vi "load_ltrace.vi"(7 "Progress":refnum<vi>, 8 "error in":errorcluster, 10 "File path":path) -> (0 "error out":errorcluster, 2 "File index":T1[](array[typedef]) {"Timestamp" format="%<%.3X>T"}, 4 "Out of order":i32, 5 "Flag names":string[](array[string]), 6 "Missing":i32)   [LabVIEW 2013]
uses:
  ltrace_index.ctl
panel:
  # "Sequence number checking"
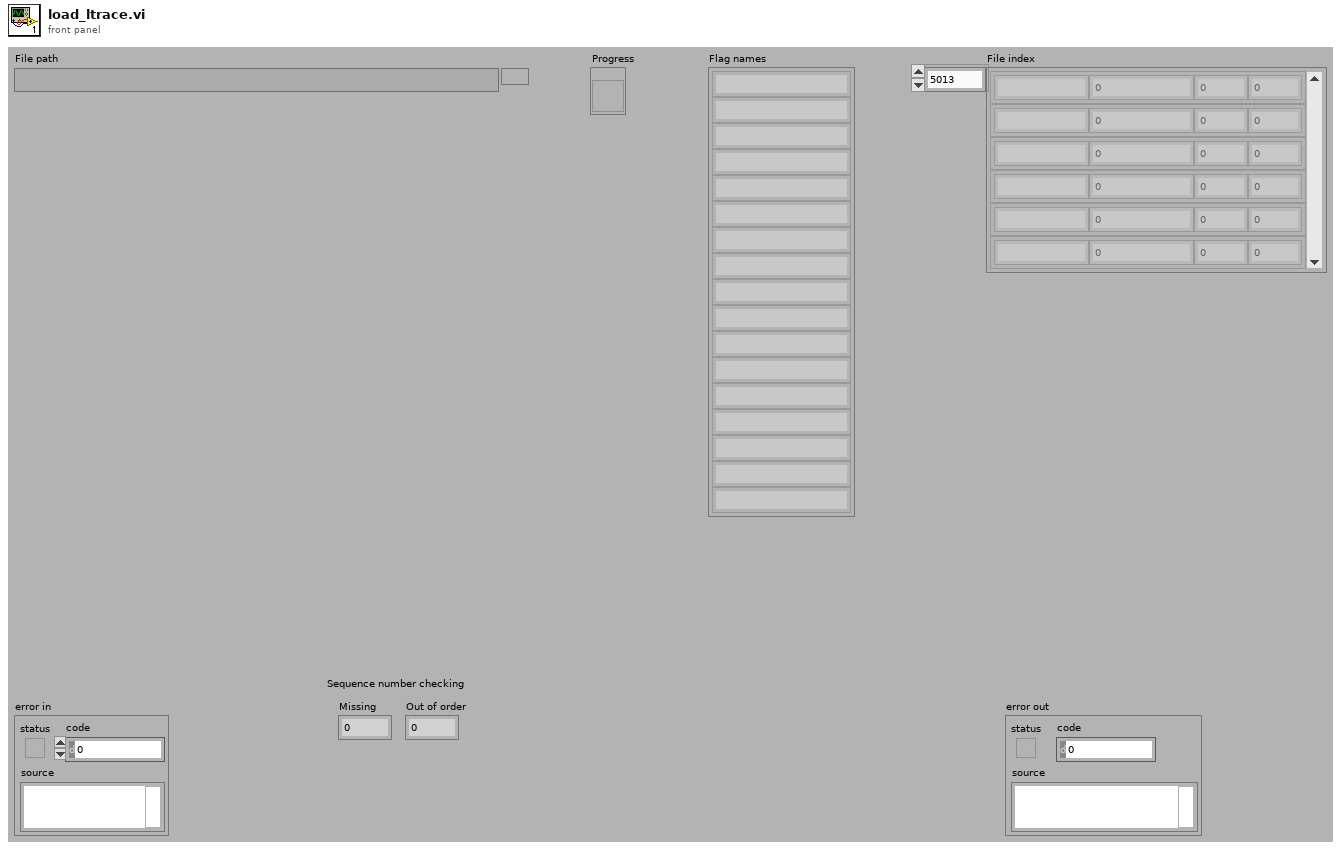
[diagram p1: front panel]
types:
  T1 = typedef "ltrace_index.ctl" = cluster{"Timestamp":timestamp, "Offset":i64, "Sequence":u32, "Flags":u32}
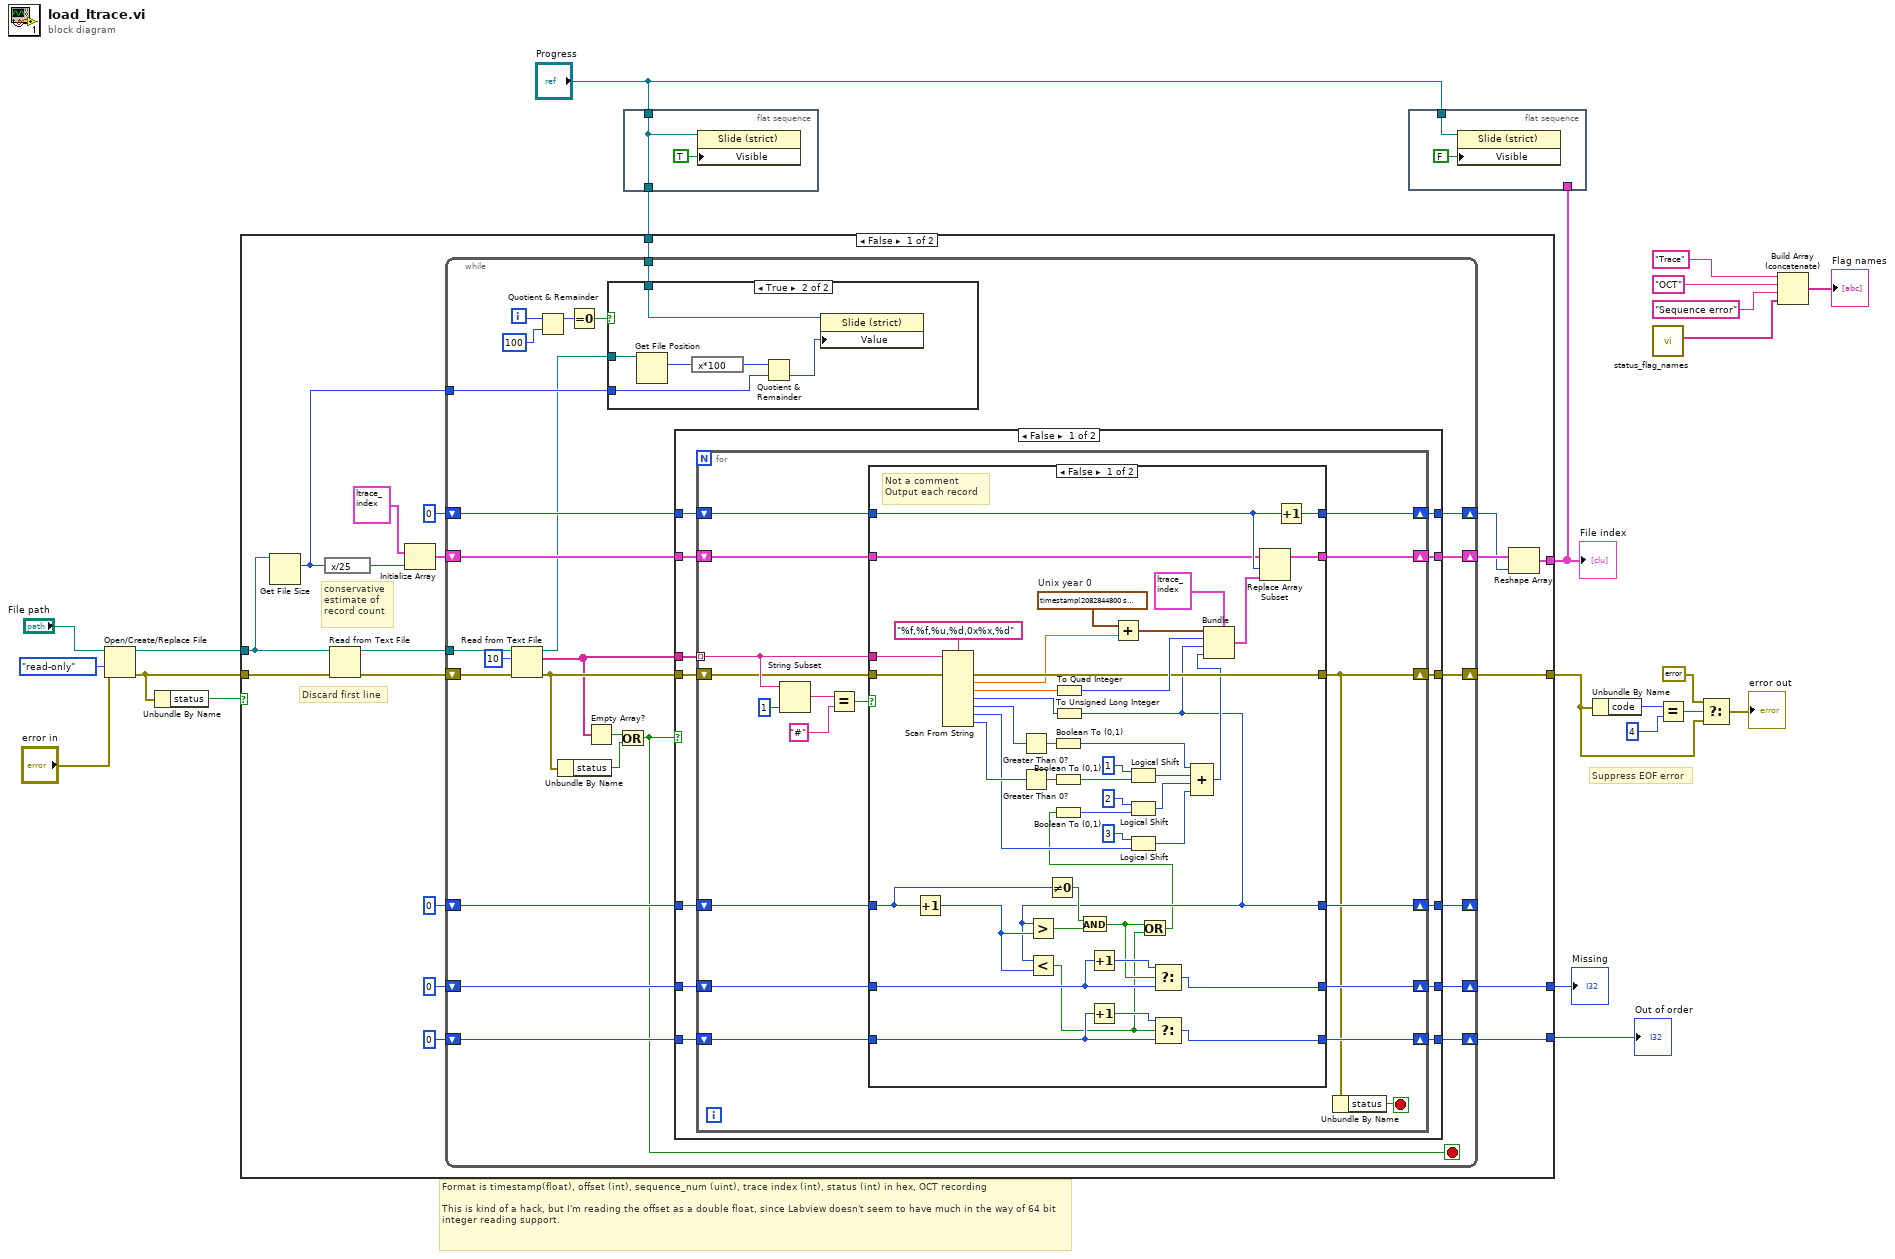
[diagram p0: block diagram]
diagram:
  # "Suppress EOF error"
  # "Format is timestamp(float), offset (int), sequence_num (uint), trace index (int), status (int) in hex, OCT recording\n\nThis is kind of a hack, but I'm reading the offset as a double float, since Labview doesn't seem to have much in the way of 64 bit integer reading support."
  n1 = Open/Create/Replace File(file path (use dialog)="File path", error in="error in", access (0:read/write)=enum16{"read/write", "read-only", "write-only"}."read-only") -> (refnum out=w14:refnum<file>, error out=w19:errorcluster)  [unwired: 3 in, 1 out]
  n2 = Unbundle By Name(w19) -> ("status"=w20:bool)
  n3 = case shown="False" w20 {
    tunnel: w19 -> [w25 w162]
    tunnel: w14 -> [w26 _]
    tunnel: [w33 _] -> w1
    tunnel: [w32 _] -> w2
    tunnel: [w31 _] -> w15
    tunnel: w17 -> [w29 _]
    tunnel: [w27 w162] -> w10
    frame False {
      # "Discard first line"
      # "conservative\nestimate of \nrecord count"
      n4 = Get File Size(file=w26) -> (size (in bytes)=w28:i64)  [unwired: 1 in, 2 out]
      n5 = expression code="x/25"(w28) -> (w30:i64)
      n6 = Read from Text File(file (use dialog)=w26, error in=w25) -> (refnum out=w23:refnum<file>, error out=w24:errorcluster)  [unwired: 2 in, 2 out]
      n7 = Initialize Array(T1 {"Timestamp"=timestamp(0 s since 1904-01-01), "Offset"=0, "Sequence"=0, "Flags"=0} ("output cluster"), w30) -> (w41:T1[])
      n8 = while {
        shift-right: [w58] -> w39
        shift-left: w41 -> [w59]
        shift-right: [w66] -> w38
        shift-left: 0 ("output 3") -> [w67]
        shift-right: [w65] -> _
        shift-left: u32 0 ("unsigned 32bit integer") -> [w64]
        shift-right: [w60] -> w32
        shift-left: 0 ("output 5") -> [w63]
        shift-right: [w61] -> w33
        shift-left: 0 ("output 5") -> [w62]
        tunnel: w29 -> [w56]
        tunnel: w28 -> [w55]
        tunnel: w23 -> [w54]
        shift-right: [w51] -> w27
        shift-left: w24 -> [w53]
        i -> [w57]
        stop <- w46 stop-if-true
        n9 = Read from Text File(file (use dialog)=w54, count=10, error in=w53) -> (refnum out=w42:refnum<file>, text=w49:string[], error out=w52:errorcluster)  [unwired: 1 in, 1 out]
        n10 = Quotient & Remainder(x=w57, y=100) -> (x-y*floor(x/y)=w43:i32)  [unwired: 1 out]
        n11 = Unbundle By Name(w52) -> ("status"=w47:bool)
        n12 = Equal To 0?(x=w43) -> (x = 0?=w44:bool)
        n13 = Empty Array?(array=w49) -> (empty?=w48:bool)
        n14 = case shown="True" w44 {
          tunnel: w56 -> [_ w73]
          tunnel: w42 -> [_ w72]
          tunnel: w55 -> [_ w69]
          frame False {
          }
          frame True {
            n15 = Get File Position(7:w72) -> (2:w71:i64)  [unwired: 1 in, 2 out]
            n16 = expression code="x*100"(w71) -> (w70:i64)
            n17 = Quotient & Remainder(x=w70, y=w69) -> (floor(x/y)=w68:i64)  [unwired: 1 out]
            n18 = property class="Slide (strict)"(reference=w73, "Value"=w68) -> ()  [unwired: 1 in, 2 out]
          }
        }
        n19 = Or(x=w48, y=w47) -> (x .or. y?=w46:bool)
        n20 = case shown="False" w46 {
          tunnel: w67 -> [w86 w156]
          tunnel: [w85 w156] -> w66
          tunnel: [w84 w160] -> w65
          tunnel: w64 -> [w83 w160]
          tunnel: w63 -> [w82 w159]
          tunnel: w62 -> [w81 w158]
          tunnel: [w80 w158] -> w61
          tunnel: [w79 w159] -> w60
          tunnel: w59 -> [w78 w157]
          tunnel: [w77 w157] -> w58
          tunnel: w49 -> [w76 _]
          tunnel: w52 -> [w75 w161]
          tunnel: [w74 w161] -> w51
          frame False {
            n21 = for {
              tunnel: w76 -> [w90] mode=indexing
              shift-right: [w101] -> w84
              shift-left: w83 -> [w100]
              shift-right: [w96] -> w79
              shift-left: w82 -> [w99]
              shift-right: [w97] -> w80
              shift-left: w81 -> [w98]
              shift-right: [w87] -> w74
              shift-left: w75 -> [w89]
              shift-right: [w102] -> w85
              shift-left: w86 -> [w103]
              shift-right: [w91] -> w77
              shift-left: w78 -> [w92]
              stop <- w88 stop-if-true
              n22 = String Subset(string=w90, length (rest)=1 ("length (rest)")) -> (substring=w95:string)  [unwired: 1 in]
              n23 = Equal?(x=w95, y="#") -> (x = y?=w93:bool)
              n24 = case shown="False" w93 {
                tunnel: w90 -> [w149 _]
                tunnel: w103 -> [w147 w155]
                tunnel: [w148 w155] -> w102
                tunnel: [w114 w152] -> w101
                tunnel: w100 -> [w146 w152]
                tunnel: w99 -> [w143 w154]
                tunnel: w98 -> [w141 w153]
                tunnel: [w140 w153] -> w97
                tunnel: [w139 w154] -> w96
                tunnel: w92 -> [w119 w151]
                tunnel: [w118 w151] -> w91
                tunnel: w89 -> [w117 w150]
                tunnel: [w116 w150] -> w87
                frame False {
                  w105 = timestamp(2082844800 s since 1904-01-01)  # Unix year 0
                  # "Not a comment\nOutput each record"
                  n25 = Increment(x=w146) -> (x+1=w145:u32)
                  n26 = Scan From String(format string="%f,%f,%u,%d,0x%x,%d", input string=w149, error in=w117) -> (error out=w116:errorcluster, output 1=w106:dbl, output 2=w132:dbl, output 3=w130:u32, output 4=w134:i32, output 5=w128:u32, output 6=w133:i32)  [unwired: 7 in, 2 out]
                  n27 = Greater Than 0?(x=w134) -> (x > 0?=w125:bool)
                  n28 = Greater Than 0?(x=w133) -> (x > 0?=w126:bool)
                  n29 = Not Equal To 0?(x=w146) -> (x != 0?=w137:bool)
                  n30 = Boolean To (0,1)(Boolean=w125) -> (0, 1=w122:i16)
                  n31 = Boolean To (0,1)(Boolean=w126) -> (0, 1=w123:i16)
                  n32 = To Quad Integer(1:w132) -> (0:w131:i64)
                  n33 = To Unsigned Long Integer(number=w130) -> (unsigned 32bit integer=w114:u32)
                  n34 = Greater?(x=w114, y=w145) -> (0:w138:bool)
                  n35 = Less?(x=w114, y=w145) -> (x < y?=w112:bool)
                  n36 = And(x=w137, y=w138) -> (x .and. y?=w113:bool)
                  n37 = Increment(x=w143) -> (x+1=w144:i32)
                  n38 = Increment(x=w141) -> (x+1=w142:i32)
                  n39 = Add(x=w105, y=w106) -> (x+y=w107:timestamp)
                  n40 = Logical Shift(y=i8 1, x=w123) -> (x << y=w121:i16)
                  n41 = Logical Shift(y=i8 3, x=w128) -> (x << y=w120:u32)
                  n42 = Or(x=w113, y=w112) -> (x .or. y?=w108:bool)
                  n43 = Boolean To (0,1)(Boolean=w108) -> (0, 1=w111:i16)
                  n44 = Logical Shift(y=i8 2, x=w111) -> (x << y=w109:i16)
                  n45 = Select(t=w144, s=w113, f=w143) -> (s? t:f=w139:i32)
                  n46 = Select(t=w142, s=w112, f=w141) -> (s? t:f=w140:i32)
                  n47 = Compound Arithmetic op=ADD(w122, w121, w109, w120) -> (w115:u32)
                  n48 = Bundle(cluster=T1 {"Timestamp"=timestamp(0 s since 1904-01-01), "Offset"=0, "Sequence"=0, "Flags"=0} ("output cluster"), "Timestamp"=w107, "Offset"=w131, "Sequence"=w114, "Flags"=w115) -> (w136:T1)
                  n49 = Replace Array Subset(array=w119, new element=w136, index=w147) -> (w118:T1[])
                  n50 = Increment(x=w147) -> (x+1=w148:i32)
                }
                frame True {
                  # "Comment"
                }
              }
              n51 = Unbundle By Name(w87) -> ("status"=w88:bool)
            }
          }
          frame True {
          }
        }
      }
      n52 = Reshape Array(w39, w38) -> (w31:T1[])
    }
    frame True {
    }
  }
  "Missing" <- w2
  "Out of order" <- w1
  "File index" <- w15
  n53 = flat-sequence {
    tunnel: "Progress" -> [w164]
    tunnel: [w164] -> w17
    frame #0 {
      n54 = property class="Slide (strict)"(reference=w164, "Visible"=TRUE) -> ()  [unwired: 1 in, 2 out]
    }
  }
  n55 = flat-sequence {
    tunnel: "Progress" -> [w166]
    tunnel: w15 -> [_]
    frame #0 {
      n56 = property class="Slide (strict)"(reference=w166, "Visible"=FALSE) -> ()  [unwired: 1 in, 2 out]
    }
  }
  n57 = Unbundle By Name(w10) -> ("code"=w13:i32)
  n58 = call "status_flag_names.vi"() -> ("Names"=w7:string[])  [unwired: 11 in]
  n59 = Equal?(x=w13, y=4 ("code")) -> (x = y?=w11:bool)
  n60 = Select(t=errorcluster {"status"=FALSE, "code"=0, "source"=""}, s=w11, f=w10) -> (s? t:f=→"error out":errorcluster)
  n61 = Build Array (concatenate)("Trace", "OCT", "Sequence error", w7) -> (→"Flag names":string[])
